vi "VCS Get Homing State.vi"(8 "error in (no error)":errorcluster, 11 "axis in":cluster{"keyHandle":u32, "nodeId":u16}={"keyHandle"=0, "nodeId"=1}) -> (0 "error out":errorcluster, 1 "homingError":i32, 2 "homingAttained":i32, 3 "axis out":cluster{"keyHandle":u32, "nodeId":u16}={"keyHandle"=0, "nodeId"=1})   [LabVIEW 2010]
doc: "The VI <B>VCS Get Homing State</B> returns the states if the homing position is attained and if an homing error is occurred."
uses:
  Resources/EposCmd.dll
  Resources/EposCmd64.dll
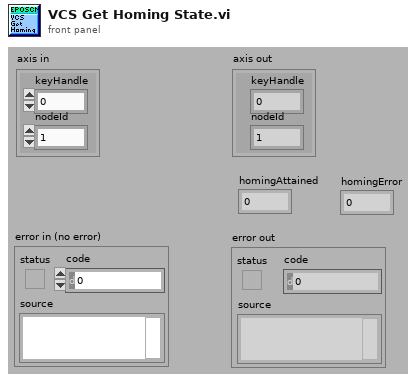
[diagram p1: front panel]
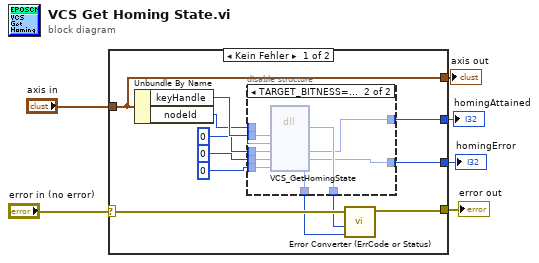
[diagram p0: block diagram]
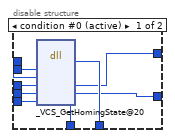
[diagram p2: hidden frame]
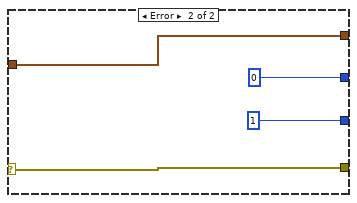
[diagram p3: hidden frame]
diagram:
  n1 = case shown="Kein Fehler" "error in (no error)" {
    selector: "error in (no error)" -> [w18 w40]
    tunnel: [w17 w40] -> w5
    tunnel: [w11 0 ("pTargetReached")] -> w4
    tunnel: "axis in" -> [w14 w39]
    tunnel: [w14 w39] -> w2
    tunnel: [w7 1 ("pTargetReached")] -> w1
    frame No Error {
      n2 = Unbundle By Name(w14) -> ("keyHandle"=w16:u32, "nodeId"=w15:u16)
      n3 = disable-structure shown="TARGET_BITNESS==64" {
        disable-tunnel: w16 -> [w27 w36]
        disable-tunnel: w15 -> [w26 w35]
        disable-tunnel: 0 ("pHomingAttained") -> [w25 w34]
        disable-tunnel: [w24 w33] -> w12
        disable-tunnel: [w23 w32] -> w11
        disable-tunnel: 0 ("pHomingError") -> [w22 w31]
        disable-tunnel: u32 0 ("pErrorCode") -> [w21 w30]
        disable-tunnel: [w20 w29] -> w8
        disable-tunnel: [w19 w28] -> w7
        frame condition #0 (active) {
          n4 = dll-call lib="C:/Sources/LabView/maxon EPOS/Resources/EposCmd.*" fn="_VCS_GetHomingState@20" ("EposCmd.dll:_VCS_GetHomingState@16")("KeyHandle"=w27, "NodeId"=w26, "pHomingAttained"=w25, "pHomingError"=w22, "pErrorCode"=w21) -> (w24:i32, "pHomingAttained"=w23:i32, "pHomingError"=w19:i32, "pErrorCode"=w20:u32)  [unwired: 5 in, 2 out]
        }
        frame condition #1 {
          n5 = dll-call lib="C:/setup/Resources/EposCmd64.*" fn="VCS_GetHomingState" ("EposCmd.dll:_VCS_GetHomingState@16")("KeyHandle"=w36, "NodeId"=w35, "pHomingAttained"=w34, "pHomingError"=w31, "pErrorCode"=w30) -> ("Rückgabetyp"=w33:i32, "pHomingAttained"=w32:i32, "pHomingError"=w28:i32, "pErrorCode"=w29:u32)  [unwired: 5 in, 2 out]
        }
      }
      n6 = call "Error Converter (ErrCode or Status).vi"("error code"=w8, "return type"=w12, "error in (no error)"=w18) -> ("error out"=w17:errorcluster)  [unwired: 7 in]
    }
    frame Error {
    }
  }
  "homingAttained" <- w4
  "error out" <- w5
  "axis out" <- w2
  "homingError" <- w1
